vi "Update channels.vi"(8 "error in (no error)":errorcluster, 11 "AOTF in":refnum<class "AOTF.lvclass">) -> (0 "error out":errorcluster, 3 "AOTF out":refnum<class "AOTF.lvclass">)   [LabVIEW 2012, in "AOTF.lvclass"]
uses:
  AOTF.lvclass
  AOTF.lvclass/AOTF.ctl
  <vilib>/DAQmx/write.llb/DAQmx Write (Digital U8 1Chan 1Samp).vi
  <vilib>/DAQmx/write.llb/DAQmx Write (Analog DBL 1Chan 1Samp).vi
  <vilib>/DAQmx/miscellaneous.llb/DAQmx Fill In Error Info.vi
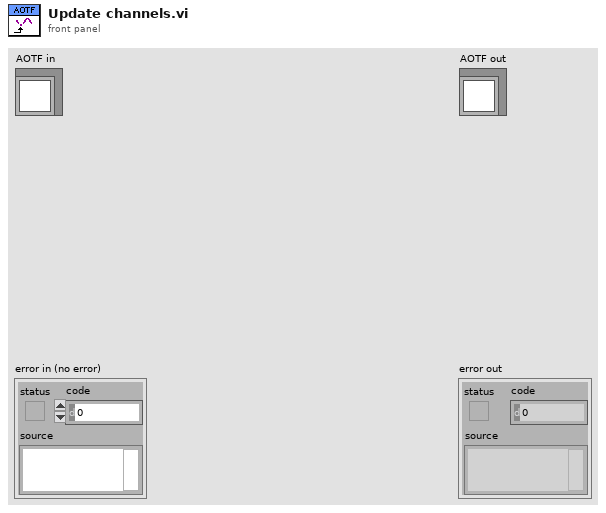
[diagram p1: front panel]
types:
  T1 = typedef "AOTF.lvclass/laser line ring.ctl" = u8
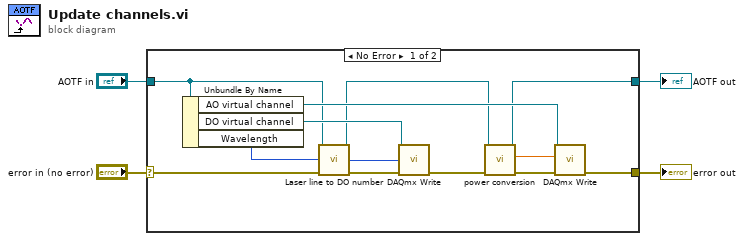
[diagram p0: block diagram]
diagram:
  n1 = case shown="No Error" "error in (no error)" {
    selector: "error in (no error)" -> [w10 w19]
    tunnel: [w17 w19] -> w3
    tunnel: [w14 w18] -> w1
    tunnel: "AOTF in" -> [w8 w18]
    frame No Error {
      n2 = Unbundle By Name(w8) -> ("AO virtual channel"=w16:refnum<k21>, "DO virtual channel"=w15:refnum<k21>, "Wavelength"=w6:T1)
      n3 = call-dynamic "Laser line to DO number.vi"("error in (no error)"=w10, "Wavelength"=w6, "AOTF in"=w8) -> ("error out"=w9:errorcluster, "DO number"=w5:u8, "AOTF out"=w7:refnum<class "AOTF.lvclass">)  [unwired: 6 in]
      n4 = call-poly <vilib>:"DAQmx Write.vi"("task/channels in"=w15, "data"=w5, "error in"=w9) -> ("error out"=w13:errorcluster)  [unwired: 10 in, 2 out]
      n5 = call-dynamic "power conversion.vi"("error in (no error)"=w13, "AOTF in"=w7) -> ("error out"=w12:errorcluster, "Power voltage out"=w11:dbl, "AOTF out"=w14:refnum<class "AOTF.lvclass">)  [unwired: 7 in]
      n6 = call-poly <vilib>:"DAQmx Write.vi"("task/channels in"=w16, "data"=w11, "error in"=w12) -> ("error out"=w17:errorcluster)  [unwired: 10 in, 2 out]
    }
    frame Error {
    }
  }
  "error out" <- w3
  "AOTF out" <- w1
